vi "Auton #3 one green bin.vi"   [LabVIEW 2014]
uses:
  Robot Global Data.vi
  <vilib>/Rock Robotics/WPI/RobotDrive/WPI_RobotDriveGetSetRefNum.vi
  <vilib>/Rock Robotics/WPI/RobotDrive/WPI_RobotDriveMecanumDrive_Cartesian.vi
types:
  T1 = enum16{"Position Bottom", "Off", "Hold", "Jog Down", "Jog Up", "Position Top", ""}
  T2 = typedef "WPI_RobotDriveDevRef.ctl" = cluster{"DevStatus":errorcluster, "Motors[]":T3[], "Square Inputs":bool, "Max Output":dbl}
  T3 = typedef "WPI_MotorControlDeviceRef.ctl" = cluster{"DeviceStatus":errorcluster, "Type":T4, "PWM":cluster{"Controller":T5, "PWM Channel":T6, "DeadBand":T7}, "CAN":cluster{"Device Number":u8, "Control Mode":T8, "Semaphore":T9, "Max Vout":dbl, "TalonSRX Control Mode":T10}, "Invert":bool, "TransformRef":T11, "InvTransformRef":T11}
  T4 = typedef "WPI_MotorControlType.ctl" = enum16{"PWM", "CAN", "CANTalonSRX"}
  T5 = typedef "FPGA_TypedefDigitalModule.ctl" = enum16{"Controller 1"}
  T6 = typedef "FPGA_DIOPWMChannel.ctl" = enum8{"PWM 0", "PWM 1", "PWM 2", "PWM 3", "PWM 4", "PWM 5", "PWM 6", "PWM 7", "PWM 8", "PWM 9", "PWM MXP 0", "PWM MXP 1", "PWM MXP 2", "PWM MXP 3", "PWM MXP 4", "PWM MXP 5", "PWM MXP 6", "PWM MXP 7", "PWM MXP 8", "PWM MXP 9", "Invalid"}
  T7 = typedef "WPI_PWMDeadband.ctl" = cluster{"Name":string, "maxPositivePwm":i32, "minPositivePwm":i32, "centerPwm":i32, "maxNegativePwm":i32, "minNegativePwm":i32, "angularRange":u16}
  T8 = typedef "WPI_CANJaguar_ControlMode.ctl" = enum8{"Percent VBus", "Current", "Speed", "Position", "Voltage"}
  T9 = typedef "Semaphore RefNum" = refnum<k1>
  T10 = typedef "WPI_CANTalonSRX_APIControlMode.ctl" = enum8{"Percent VBus", "Speed", "Position", "Slave", "Unchanged / Invalid"}
  T11 = typedef "WPI_PWMTransform_ConPane.ctl" = refnum<vi>
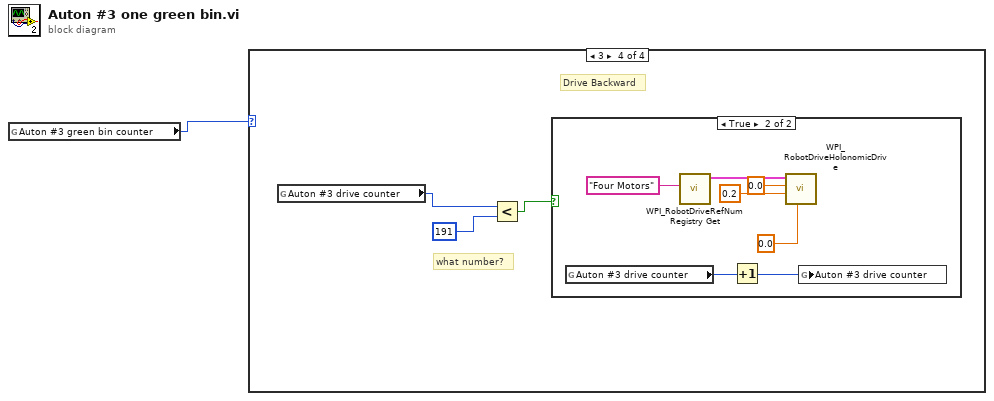
[diagram p0: block diagram]
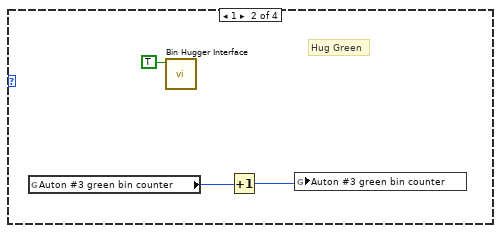
[diagram p3: hidden frame]
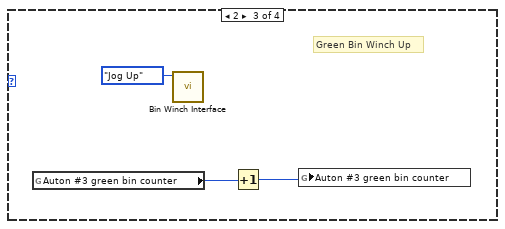
[diagram p4: hidden frame]
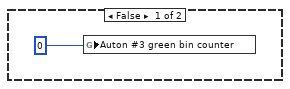
[diagram p5: hidden frame]
diagram:
  n1 = global read "Robot Global Data.vi" "Auton #3 green bin counter"() -> (w1:i8)
  n2 = case shown="3" w1 {
    frame 0, Default {
    }
    frame 1 {
      # "Hug Green"
      n3 = global read "Robot Global Data.vi" "Auton #3 green bin counter"() -> (w3:i8)
      n4 = call "Bin Hugger Interface.vi"("Close Bin Hugger"=TRUE) -> ()  [unwired: 10 in, 1 out]
      n5 = Increment(x=w3) -> (x+1=w2:i8)
      n6 = global write "Robot Global Data.vi" "Auton #3 green bin counter"(w2) -> ()
    }
    frame 2 {
      # "Green Bin Winch Up"
      n7 = global read "Robot Global Data.vi" "Auton #3 green bin counter"() -> (w6:i8)
      n8 = call "Bin Winch Interface.vi"("Winch Command"=T1."Jog Up") -> ()  [unwired: 11 in]
      n9 = Increment(x=w6) -> (x+1=w5:i8)
      n10 = global write "Robot Global Data.vi" "Auton #3 green bin counter"(w5) -> ()
    }
    frame 3 {
      # "Drive Backward"
      # "what number?"
      n11 = global read "Robot Global Data.vi" "Auton #3 drive counter"() -> (w9:i16)
      n12 = Less?(x=w9, y=i16 191) -> (x < y?=w10:bool)
      n13 = case shown="True" w10 {
        frame False {
          n14 = global write "Robot Global Data.vi" "Auton #3 green bin counter"(i16 0 ("Auton #3 drive counter")) -> ()
        }
        frame True {
          n15 = global read "Robot Global Data.vi" "Auton #3 drive counter"() -> (w13:i16)
          n16 = call <vilib>:"WPI_RobotDriveRefNum Registry Get.vi"("refnum name"="Four Motors") -> ("RobotDriveDevRef"=w17:T2)  [unwired: 1 in, 9 out]
          n17 = Increment(x=w13) -> (x+1=w12:i16)
          n18 = call-poly <vilib>:"WPI_RobotDriveHolonomicDrive.vi"("Rotation"=0.0, "Y"=0.2, "X"=0.0, "RobotDriveDevRef"=w17) -> ()  [unwired: 5 in, 3 out]
          n19 = global write "Robot Global Data.vi" "Auton #3 drive counter"(w12) -> ()
        }
      }
    }
  }
